vi "export Complex Data 1D.vi"(4 "error in (no error)":errorcluster, 5 "Export File":path, 6 "Data 2D Export Format Selection":T1, 7 "Data in":refnum<class "Data.lvclass">) -> (0 "error out":errorcluster, 3 "Data out":refnum<class "Data.lvclass">)   [LabVIEW 2018]
uses:
  SpectralRadar/LabVIEW/2012/user.lib/SpectralRadar.llb/Data.lvclass
  SpectralRadar/LabVIEW/2012/user.lib/SpectralRadar.llb/Data 2D Export Format Selection.ctl
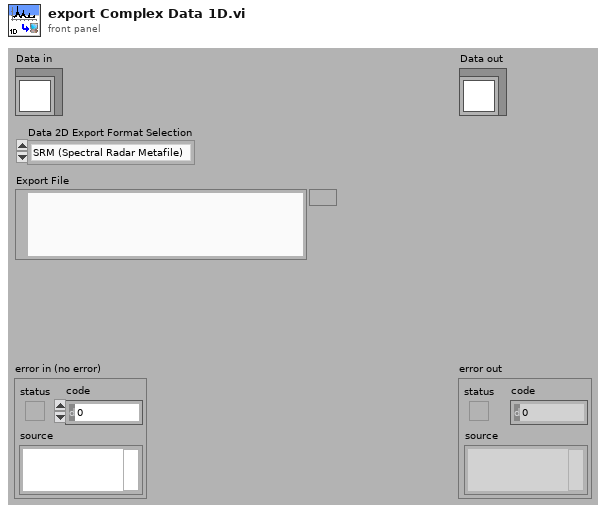
[diagram p1: front panel]
types:
  T1 = typedef "Data.lvclass/Data 2D Export Format Selection.ctl" = enum16{"SRM (Spectral Radar Metafile)", "RAW", "TXT", "CSV", "TXT Table"}
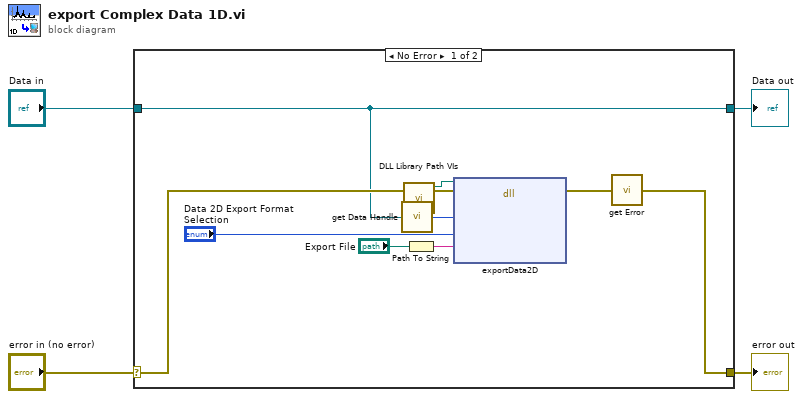
[diagram p0: block diagram]
diagram:
  n1 = case shown="No Error" "error in (no error)" {
    selector: "error in (no error)" -> [w13 w15]
    tunnel: [w6 w15] -> w3
    tunnel: [w11 w14] -> w1
    tunnel: "Data in" -> [w11 w14]
    frame No Error {
      n2 = call "get Data Handle.vi"("Data"=w11) -> ("Handle"=w10:u64)
      n3 = call "DLL Library Path VIs.vi"() -> ("SpectralRadarDLL"=w5:path)  [unwired: 8 in, 3 out]
      n4 = Path To String(path="Export File") -> (string=w9:string)
      n5 = dll-call lib="C:/Project/SerialSectOCT - FFT GPU/SerialSectOCT/Labview Software/DLL/SpectralRadar.dll" fn="exportData2D"(path in=w5, error in=w13, "Data Handle"=w10, "Export Format"="Data 2D Export Format Selection", "File Name"=w9) -> (error out=w7:errorcluster)  [unwired: 5 in, 1 out]
      n6 = call "get Error.vi"("error in (no error)"=w7) -> ("error out"=w6:errorcluster)
    }
    frame Error {
    }
  }
  "error out" <- w3
  "Data out" <- w1
